vi "Text-Parse String Fields.vi"(0 "String":string, 11 "Separator":string=":") -> (4 "Fields":string[](array[string]), 6 "element":string, 8 "element 2":string, 10 "element 3":string, 14 "Number of fields":u32, 15 "element 4":string)   [LabVIEW 2020]
doc: "Returns an array of Fields parsed out of String. Fields are separated by the string Separator (default \":\")."
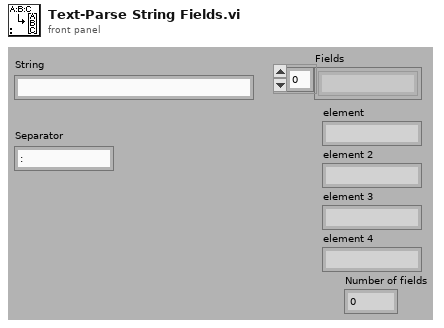
[diagram p1: front panel]
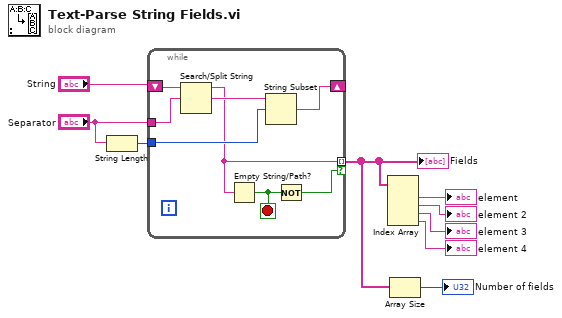
[diagram p0: block diagram]
diagram:
  n1 = String Length(string="Separator") -> (length=w6:i32)
  n2 = while {
    shift-right: [w15] -> _
    shift-left: "String" -> [w17]
    tunnel: "Separator" -> [w14]
    tunnel: w6 -> [w13]
    tunnel: [w12] -> w5 mode=indexing if=w10
    stop <- w11 stop-if-true
    n3 = Search/Split String(string=w17, search string/char (-)=w14) -> (substring before match=w12:string, match + rest of string=w16:string)  [unwired: 1 in, 1 out]
    n4 = Empty String/Path?(string/path=w12) -> (empty?=w11:bool)
    n5 = String Subset(string=w16, offset (0)=w13) -> (substring=w15:string)  [unwired: 1 in]
    n6 = Not(x=w11) -> (.not. x?=w10:bool)
  }
  "Fields" <- w5
  n7 = Index Array(array=w5) -> (element #1=→"element":string, element #2=→"element 2":string, element #3=→"element 3":string, element #4=→"element 4":string)  [unwired: 4 in]
  n8 = Array Size(array=w5) -> (size(s)=→"Number of fields":i32)
